vi "Create Python Orchestration Script.vi"(7 "Override Address":bool, 8 "error in":errorcluster, 9 "Default Address":string, 10 "Configuration File Name":string="orchestration.py", 11 "Filtered Config Entries":string="1737340154015584000\ttest\tCreate\tTemplatePlugin.0.2.3.lvlibp:TemplatePlugin.lvclass\t<version> 0.2.3.0\t<loader> Default_LabVIEW\t\n1737340198541890000\ttest\tConfigure\t{\"Common\":{\"Period (s)\":0.001,\"Offset (us)\":0,\"ClockID\":0,\"Priority\":101,\"Processor\":-2},\"Step\":100}\n1737340326509796000\tlovingit6\tCreate\tCIFCorePlugin.0.1.2.lvlibp:CIFCorePlugin.lvclass\t<version> 0.1.2.0\t<loader> Default_LabVIEW\t\n1737340326559504000\tchannelme\tCreate\tTemplatePlugin.0.2.3.lvlibp:TemplatePlugin.lvclass\t<version> 0.2.3.0\t<loader> Default_LabVIEW\t\n1737340326827852000\tchannelme\tConnect\t<publisher> channelme/doubleout <subscriber> channelme/doublein1 <data> \n1737340326835711000\tchannelme\tConfigure\t{\"Common\":{\"Period (s)\":0.001,\"Offset (us)\":0,\"ClockID\":0,\"Priority\":101,\"Processor\":-2},\"Step\":100}\n1737340327017380000\tlovingit6\tRun\n") -> (0 "error out":errorcluster, 2 "Orchestration File Path":path, 3 "Python Orchestration File":string)   [LabVIEW 2021, in "Python Orchestration.lvlib"]
uses:
  Python Orchestration.lvlib
  <vilib>/CIF Foundation/CIF Core/CIFUtilities/CIFConfigurationFile/typedef/Location Type.ctl
  <vilib>/CIF Foundation/CIF Core/CIFUtilities/CIFConfigurationFile/CIF Configuration File Location.vi
  <vilib>/CIF Foundation/CIF Core/CIFUtilities/CIFConfigurationFile/CIF Configuration File.lvlib
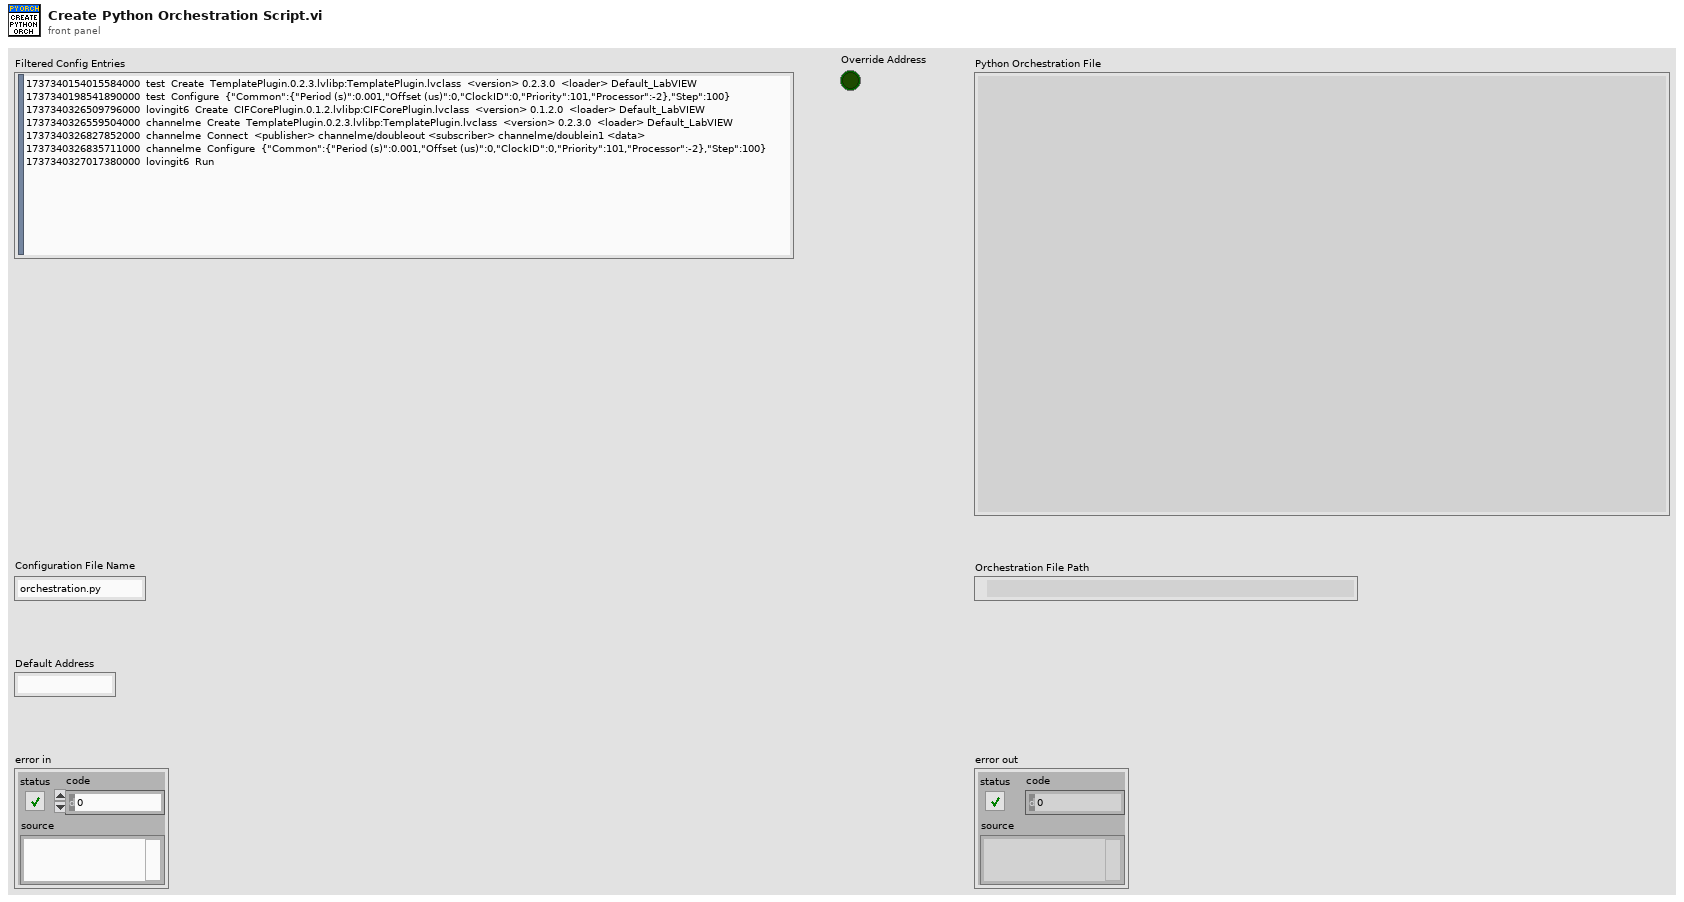
[diagram p1: front panel]
types:
  T1 = typedef "CIF Configuration File.lvlib/Location Type.ctl" = enum16{"Config File", "Manager", "Protos", "Plugins", "UI Plugins", "Logs", "Orchestrations", "Loaders"}
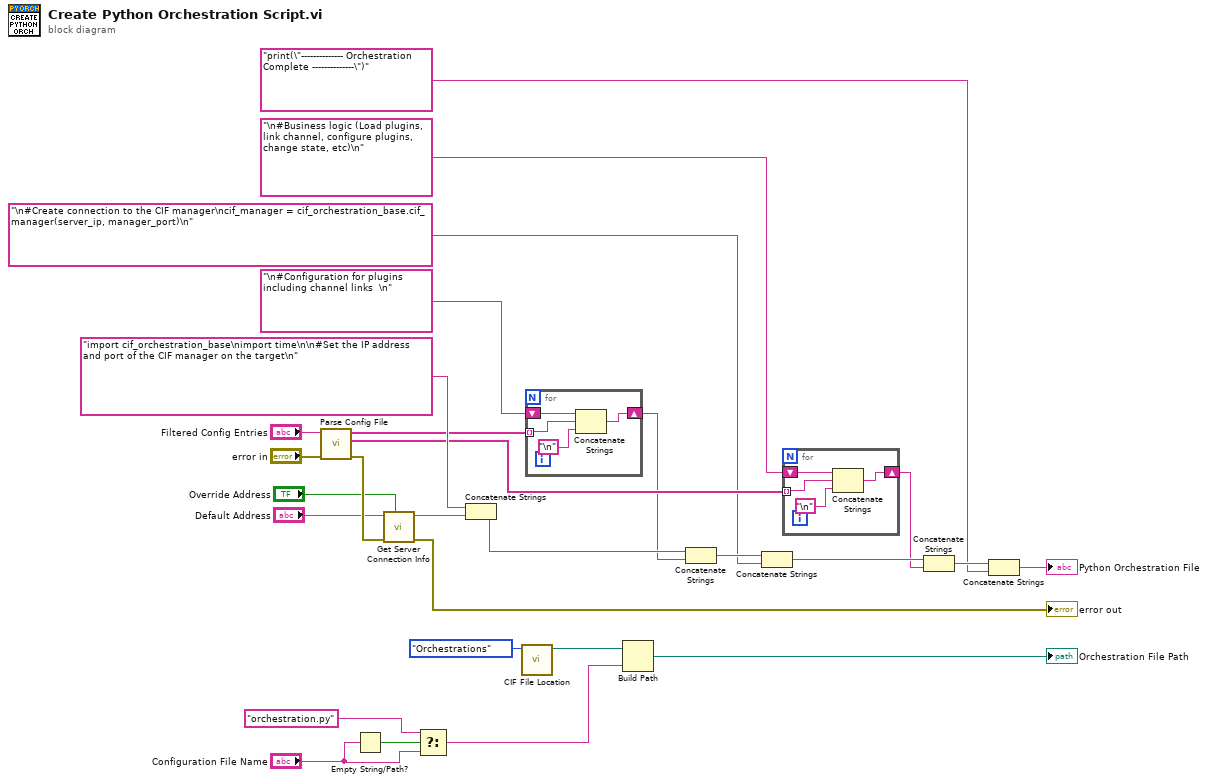
[diagram p0: block diagram]
diagram:
  n1 = call "Parse Config File.vi"("error in (no error)"="error in", "Filtered Config Entries"="Filtered Config Entries") -> ("error out"=w24:errorcluster, "Logic Entries"=w20:string[], "Configuration Entries"=w23:string[])  [unwired: 7 in]
  n2 = Empty String/Path?(string/path="Configuration File Name") -> (empty?=w6:bool)
  n3 = call "Get Server Connection Info.vi"("Override Address"="Override Address", "error in"=w24, "Default Address"="Default Address") -> ("error out"=→"error out":errorcluster, "Server Connection"=w26:string)  [unwired: 7 in]
  n4 = Select(t="orchestration.py" ("Configuration File Name 2"), s=w6, f="Configuration File Name") -> (s? t:f=w3:string)
  n5 = Concatenate Strings("import cif_orchestration_base\nimport time\n\n#Set the IP address and port of the CIF manager on the target\n", w26) -> (w19:string)
  n6 = call <vilib>:"CIF File Location.vi"("LocationType"=Location_Type."Orchestrations") -> ("Location"=w1:path)  [unwired: 10 in]
  n7 = for {
    tunnel: w23 -> [w31] mode=indexing
    shift-right: [w30] -> w11
    shift-left: "\n#Configuration for plugins including channel links  \n" -> [w32]
    n8 = Concatenate Strings(w32, w31, "\n") -> (w30:string)
  }
  n9 = Build Path(base path=w1, name or relative path=w3) -> (appended path=→"Orchestration File Path":path)
  n10 = Concatenate Strings(w19, w11) -> (w18:string)
  n11 = Concatenate Strings(w18, "\n#Create connection to the CIF manager\ncif_manager = cif_orchestration_base.cif_manager(server_ip, manager_port)\n") -> (w16:string)
  n12 = for {
    tunnel: w20 -> [w35] mode=indexing
    shift-right: [w34] -> w15
    shift-left: "\n#Business logic (Load plugins, link channel, configure plugins, change state, etc)\n" -> [w36]
    n13 = Concatenate Strings(w36, w35, "\n") -> (w34:string)
  }
  n14 = Concatenate Strings(w16, w15) -> (w14:string)
  n15 = Concatenate Strings(w14, "print(\"-------------- Orchestration Complete --------------\")") -> (→"Python Orchestration File":string)
